vi "Set Hold - Check & Resend.vi"(8 "error in (no error)":errorcluster) -> (0 "error out":errorcluster)   [LabVIEW 2016, in "IPS-120.lvlib" / "IPS-120-API.lvlib"]
uses:
  IPS-120-API.lvlib
  IPS120/Typedefs/Read Activity - Enum.ctl
  IPS-120.lvlib
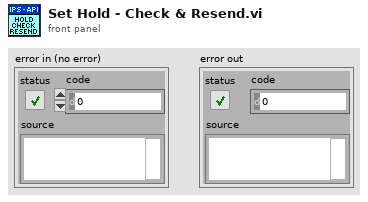
[diagram p1: front panel]
types:
  T1 = typedef "IPS-120.lvlib/Read Activity - Enum.ctl" = enum16{"Hold", "To Set Point", "To Zero", "Clamped"}
  T2 = cluster{"Hold":bool, "Clamp":bool, "To Set":bool, "To Zero":bool, "Send to IPS":bool, "PS Heat":bool}
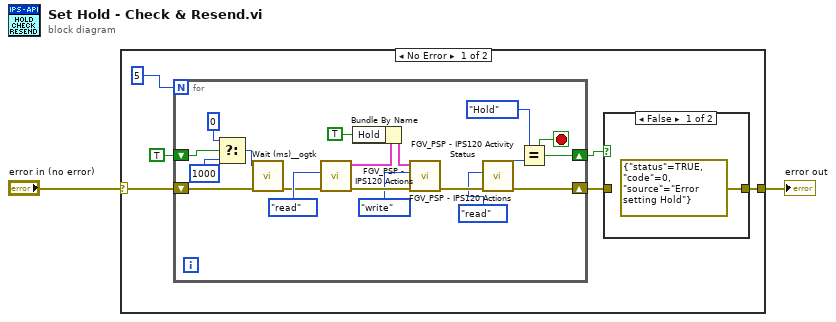
[diagram p0: block diagram]
diagram:
  n1 = case shown="No Error" "error in (no error)" {
    selector: "error in (no error)" -> [w3 w29]
    tunnel: [w4 w29] -> w2
    frame No Error {
      n2 = for {
        N: 5 -> [_]
        shift-right: [w28] -> w6
        shift-left: w3 -> [w14]
        shift-right: [w12] -> w5
        shift-left: TRUE -> [w11]
        stop <- w12 stop-if-true
        n3 = Select(t=u32 0 ("milliseconds to wait"), s=w11, f=u32 1000 ("milliseconds to wait")) -> (s? t:f=w15:u32)
        n4 = call <userlib>:"Wait (ms)__ogtk.vi"("error in (no error)"=w14, "milliseconds to wait"=w15) -> ("error out"=w13:errorcluster)  [unwired: 8 in, 1 out]
        n5 = call "FGV_PSP - IPS120 Actions.vi"("error in"=w13, "Function"=enum16{"write", "read"}."read") -> ("error out"=w24:errorcluster, "actions"=w25:T2)  [unwired: 4 in]
        n6 = Bundle By Name(cluster=w25, "Hold"=TRUE ("Send to IPS")) -> (w26:T2)
        n7 = call "FGV_PSP - IPS120 Actions.vi"("error in"=w24, "Function"=enum16{"write", "read"}."write", "actions"=w26) -> ("error out"=w27:errorcluster)  [unwired: 3 in, 1 out]
        n8 = call "FGV_PSP - IPS120 Activity Status.vi"("error in"=w27, "Function"=enum16{"write", "read"}."read") -> ("error out"=w28:errorcluster, "Activity"=w20:T1)  [unwired: 4 in]
        n9 = Equal?(x=Read_Activity_-_Enum."Hold", y=w20) -> (x = y?=w12:bool)
      }
      n10 = case shown="False" w5 {
        tunnel: w6 -> [_ w10]
        tunnel: [errorcluster {"status"=TRUE, "code"=0, "source"="Error setting Hold"} ("error in (no error)") w10] -> w4
        frame False {
        }
        frame True {
        }
      }
    }
    frame Error {
    }
  }
  "error out" <- w2
